vi "Move Forward.vi"   [LabVIEW 2016, in "LEGO-PMR.lvrbt"]
uses:
  LEGO-PMR.lvrbt
  <vilib>/NXT/Block Support/NXT_OutputPort.ctl
  <vilib>/NXT/NXTIO Xnodes/NXTIONodeSubVIs/LEGOResetMotors.vi
  <vilib>/NXT/NXTIO Xnodes/NXTIONodeSubVIs/NXTMotorSteeringOn.vi
  <vilib>/NXT/Dual Mode Library/Waits/Wait_Num.vi
  <vilib>/NXT/NXTIO Xnodes/AddressXNode/NXTIOAddress.xnode
  <vilib>/NXT/Subs/LVHSConnector.ctl
  <vilib>/NXT/NXTIO Xnodes/NXTIOXNode/NXTIO.xnode
  <vilib>/NXT/LegoClasses/BrickReference/BrickReference.lvclass
types:
  T1 = typedef "NXT_OutputPort.ctl" = u8
  T2 = typedef "LVHSConnector.ctl" = refnum<class "BrickReference.lvclass">
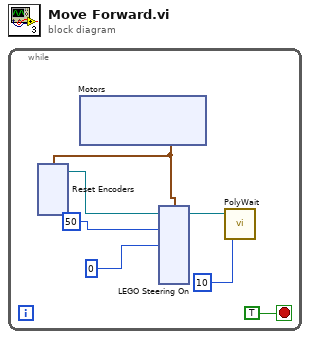
[diagram p0: block diagram]
diagram:
  n1 = while {
    stop <- TRUE stop-if-true
    n2 = xnode "Motors"() -> ("Motor"=w2:cluster{"Port":T1, "Port":T1})
    n3 = xnode "Reset Encoders"("Motors"=w2) -> ("NXT/EV3"=w1:T2)  [unwired: 1 in]
    n4 = xnode "LEGO Steering On"("Steering 1"=0, "Power 1"=50, "Motors"=w2, "NXT/EV3"=w1) -> ("NXT/EV3"=w4:T2)
    n5 = call-poly <vilib>:"PolyWait.vi"("Time (1 sec)"=10, "NXT/EV3"=w4) -> ()  [unwired: 2 in, 1 out]
  }
